vi "REV or CTRE compare.vi"() -> ()   [LabVIEW 2019]
uses:
  Motor Type.ctl
panel:
  out "CTRE Chart":cluster{dbl[unit], dbl[unit]}(graph)
  out "Rev Chart":cluster{dbl[unit], dbl[unit]}(graph)
  out "Torque 2":dbl[unit]
  out "Current 2":dbl[unit]
  out "Torque":dbl[unit]
  out "Current":dbl[unit]
  in  "CTRE":T1=enum."Neo"
  in  "REV":T1=enum."Neo"
  # "six of these\nlimited to 50A"
  # "four of these\nlimited to 75A"
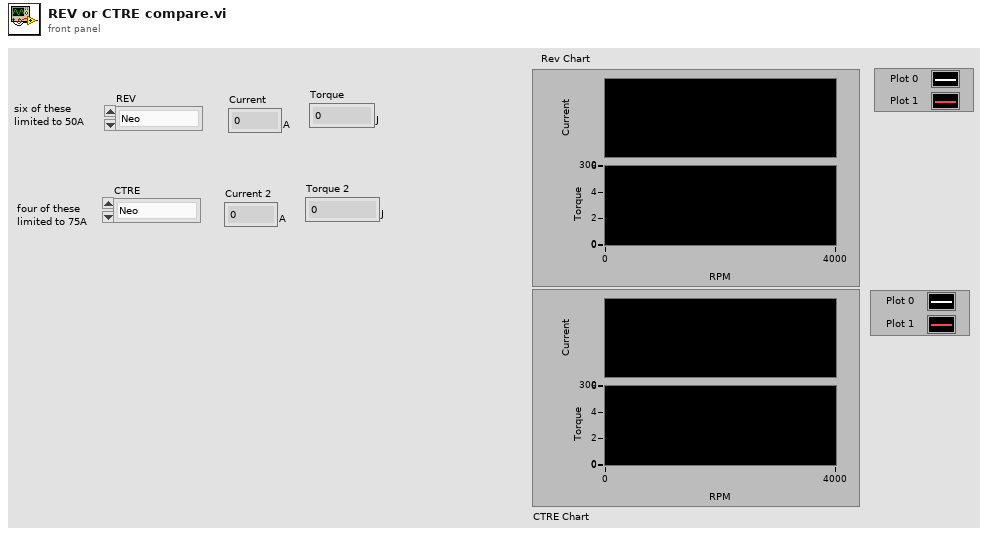
[diagram p1: front panel]
types:
  T1 = typedef "Motor Type.ctl" = enum16{"Custom", "775 pro", "CIM", "miniCIM", "Neo", "Neo 550", "Falcon 500"}
  T2 = typedef "Motor Operating Values.ctl" = cluster{"Kv":dbl[unit], "R":dbl[unit], "Kt":dbl[unit], "Breaker Size":dbl[unit]}
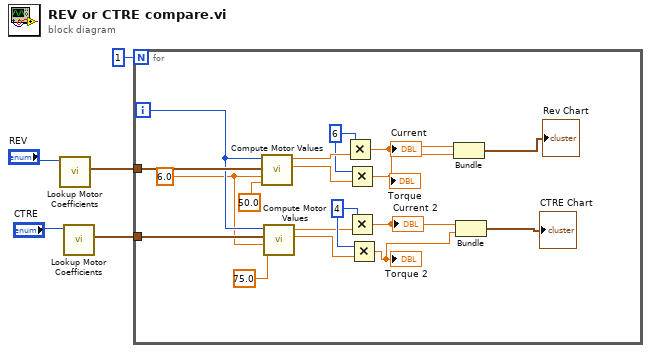
[diagram p0: block diagram]
diagram:
  n1 = call "Lookup Motor Coefficients.vi"("Motor Type"="REV") -> ("Motor Model Values"=w3:T2)  [unwired: 7 in, 3 out]
  n2 = call "Lookup Motor Coefficients.vi"("Motor Type"="CTRE") -> ("Motor Model Values"=w2:T2)  [unwired: 7 in, 3 out]
  n3 = for {
    N: 1 -> [_]
    tunnel: w3 -> [w23]
    tunnel: w2 -> [w22]
    i -> [w7]
    w6 = dbl[unit] 6.0 ("Effective Motor Voltage")
    w18 = 4
    w19 = 6
    n4 = call "Compute Motor Values.vi"("Current Limit"=dbl[unit] 50.0, "Effective Motor Voltage"=w6, "Motor Model Values"=w23, "motor speed (rpm)"=w7) -> ("Motor Torque"=w20:dbl[unit], "Current"=w21:dbl[unit])  [unwired: 4 in, 2 out]
    n5 = call "Compute Motor Values.vi"("Current Limit"=dbl[unit] 75.0, "Effective Motor Voltage"=w6, "Motor Model Values"=w22, "motor speed (rpm)"=w7) -> ("Motor Torque"=w16:dbl[unit], "Current"=w17:dbl[unit])  [unwired: 4 in, 2 out]
    n6 = Multiply(x=w19, y=w21) -> (x*y=w13:dbl[unit])
    "Current" <- w13
    n7 = Multiply(x=w19, y=w20) -> (x*y=w12:dbl[unit])
    "Torque" <- w12
    n8 = Multiply(x=w18, y=w17) -> (x*y=w11:dbl[unit])
    "Current 2" <- w11
    n9 = Multiply(x=w18, y=w16) -> (x*y=w10:dbl[unit])
    "Torque 2" <- w10
    n10 = Bundle(w13, w12) -> (→"Rev Chart":cluster{dbl[unit], dbl[unit]})  [unwired: 1 in]
    n11 = Bundle(w11, w10) -> (→"CTRE Chart":cluster{dbl[unit], dbl[unit]})  [unwired: 1 in]
  }
